vi "test_EmptyInstrumentTypeId_InitializeSessions_ReturnsError.vi"(8 "error in":errorcluster) -> (0 "error out":errorcluster, 2 "result":string, 3 "pass":bool)   [LabVIEW 2020, in "MeasurementServerTests.lvlib"]
uses:
  MeasurementServerTests.lvlib
  Helpers/Fake Session Factory/Fake Session Factory.lvclass
  da6ffb6f-c1c9-4957-84dd-e9228483c454.vi
  Runtime/Measurements/Helpers/Error Strings Global Internal.vi
  f4044373-92c1-44c4-bfbc-759c068f2270.vi
  Runtime/APIs/Session Management V1/Session Reservation/Initialize and Close Session Behavior.ctl
  Runtime/APIs/Session Management V1/Session Reservation/Session Reservation.lvclass
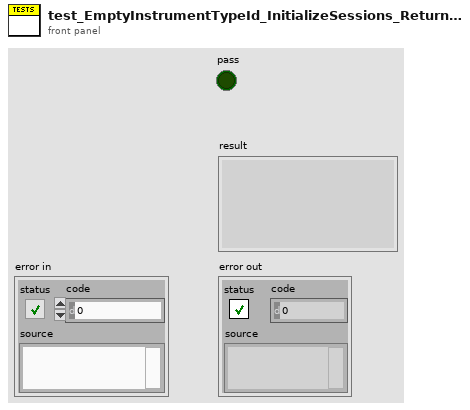
[diagram p1: front panel]
types:
  T1 = typedef "Plug-In SDK Session Management V1 API.lvlib/Session Reservation.lvclass/Initialize and Close Session Behavior.ctl" = enum16{"Auto", "Initialize and Close", "Attach and Detach", "Initialize and Detach", "Attach and Close"}
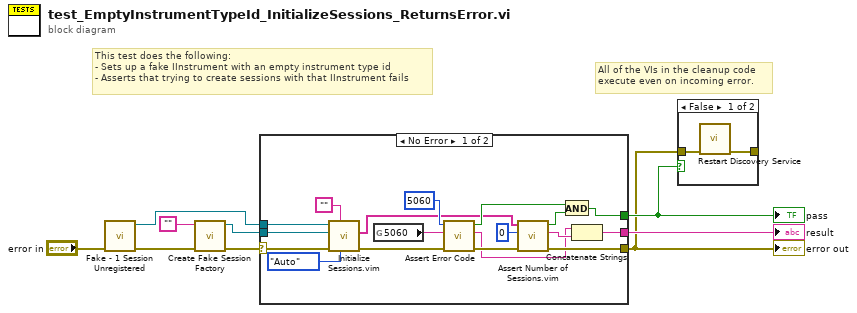
[diagram p0: block diagram]
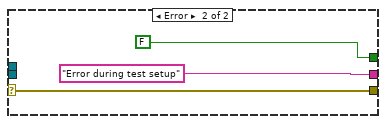
[diagram p2: hidden frame]
diagram:
  # "All of the VIs in the cleanup code\nexecute even on incoming error."
  # "This test does the following:\n- Sets up a fake IInstrument with an empty instrument type id\n- Asserts that trying to create sessions with that IInstrument fails"
  n1 = call "Fake - 1 Session Unregistered.vi"("error in"="error in") -> ("error out"=w6:errorcluster, "session reservation out"=w2:refnum<class "Session Reservation.lvclass">)  [unwired: 9 in]
  n2 = call "Create Fake Session Factory.vi"("error in"=w6, "instrument type id"="") -> ("error out"=w4:errorcluster, "fake session factory out"=w3:refnum<class "Fake Session Factory.lvclass">)  [unwired: 8 in]
  n3 = case shown="No Error" w4 {
    selector: w4 -> [w25 w28]
    tunnel: [w16 w28] -> w7
    tunnel: [w12 FALSE] -> w8
    tunnel: [w14 "Error during test setup" ("f")] -> w9
    tunnel: w3 -> [w27 _]
    tunnel: w2 -> [w26 _]
    frame No Error {
      n4 = call "Initialize Sessions.vim"("initialize and close session behavior"=Initialize_and_Close_Session_Behavior."Auto", "session type"="", "error in"=w25, "session factory"=w27, "session reservation in"=w26) -> ("error out"=w24:errorcluster, "sessions"=w11:string[])  [unwired: 3 in, 2 out]
      n5 = global read "Error Strings Global Internal.vi" "5060"() -> (w21:string)
      n6 = call "Assert Error Code.vi"("error in"=w24, "expected error description"=w21, "expected error code"=5060) -> ("error out"=w17:errorcluster, "details"=w15:string, "error code match?"=w13:bool)  [unwired: 6 in]
      n7 = call "Assert Number of Sessions.vim"("error in"=w17, "expected number of sessions"=0, "sessions"=w11) -> ("error out"=w16:errorcluster, "result"=w18:string, "pass"=w19:bool)  [unwired: 6 in]
      n8 = And(x=w13, y=w19) -> (x .and. y?=w12:bool)
      n9 = Concatenate Strings(w15, w18) -> (w14:string)
    }
    frame Error {
    }
  }
  "error out" <- w7
  "pass" <- w8
  "result" <- w9
  n10 = case shown="False" w8 {
    tunnel: w7 -> [w32 _]
    tunnel: [w31 _] -> _
    frame False {
      n11 = call "Restart Discovery Service.vi"("error in"=w32) -> ("error out"=w31:errorcluster)  [unwired: 10 in]
    }
    frame True {
    }
  }
